vi "Kikusui PLZ-Configure Input.vi"(8 "error in":errorcluster, 9 "Enable Input Short":bool, 10 "Enable Input":bool, 11 "Kikusui PLZ Setting In":T1={"VISA Resource Name"="", "Baud Rate"=19200, "Stop Bits"=20, "Wait For Read(ms)"=0} {"Stop Bits" items=["1.0"=10, "2.0"=20]; "Baud Rate" items=["2400"=2400, "4800"=4800, "9600"=9600, "19200"=19200]}) -> (0 "error out":errorcluster, 3 "Kikusui PLZ Setting Out":T1={"VISA Resource Name"="", "Baud Rate"=19200, "Stop Bits"=20, "Wait For Read(ms)"=0} {"Stop Bits" items=["1.0"=10, "2.0"=20]; "Baud Rate" items=["2400"=2400, "4800"=4800, "9600"=9600, "19200"=19200]})   [LabVIEW 2018]
doc: "Configures the input state and the input short to either on or off."
uses:
  Data Def/Kikusui PLZ-Setting.ctl
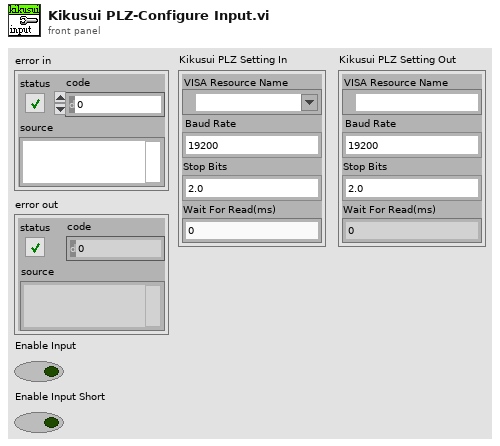
[diagram p1: front panel]
types:
  T1 = typedef "Kikusui PLZ-Setting.ctl" = cluster{"VISA Resource Name":refnum<visa-resource-name>, "Baud Rate":u32, "Stop Bits":u16, "Wait For Read(ms)":u32}
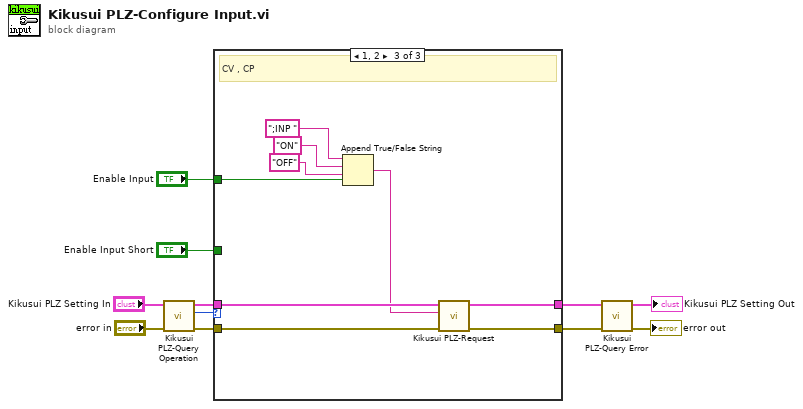
[diagram p0: block diagram]
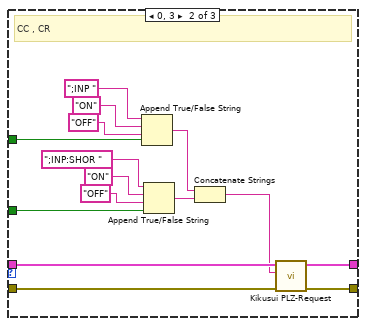
[diagram p3: hidden frame]
diagram:
  n1 = call "Kikusui PLZ-Query Operation.vi"("error in"="error in", "Kikusui PLZ Setting In"="Kikusui PLZ Setting In") -> ("error out"=w4:errorcluster, "Operation Mode"=w3:u16, "Kikusui PLZ Setting Out"=w5:T1)  [unwired: 7 in]
  n2 = case shown="1, 2" w3 {
    tunnel: w5 -> [w13 w17 w30]
    tunnel: w4 -> [w12 w18 w33]
    tunnel: "Enable Input" -> [_ w22 w34]
    tunnel: "Enable Input Short" -> [_ w21 _]
    tunnel: [w12 w15 w32] -> w9
    tunnel: [w13 w16 w31] -> w8
    frame Default {
    }
    frame 0, 3 {
      # "CC , CR"
      n3 = Append True/False String(1:w22, 2:"OFF" ("false string"), 3:"ON" ("true string"), 4:";INP " ("string (\"\")")) -> (0:w19:string)
      n4 = Append True/False String(1:w21, 2:"OFF" ("false string"), 3:"ON" ("true string"), 4:";INP:SHOR " ("string (\"\")")) -> (0:w20:string)
      n5 = Concatenate Strings(w19, w20) -> (w14:string)
      n6 = call "Kikusui PLZ-Request.vi"("error in"=w18, "Command"=w14, "Kikusui PLZ Setting In"=w17) -> ("error out"=w15:errorcluster, "Kikusui PLZ Setting Out"=w16:T1)  [unwired: 6 in, 1 out]
    }
    frame 1, 2 {
      # "CV , CP"
      n7 = Append True/False String(1:w34, 2:"OFF" ("false string"), 3:"ON" ("true string"), 4:";INP " ("string (\"\")")) -> (0:w29:string)
      n8 = call "Kikusui PLZ-Request.vi"("error in"=w33, "Command"=w29, "Kikusui PLZ Setting In"=w30) -> ("error out"=w32:errorcluster, "Kikusui PLZ Setting Out"=w31:T1)  [unwired: 6 in, 1 out]
    }
  }
  n9 = call "Kikusui PLZ-Query Error.vi"("error in"=w9, "Kikusui PLZ Setting In"=w8) -> ("error out"=→"error out":errorcluster, "Kikusui PLZ Setting Out"=→"Kikusui PLZ Setting Out":T1)  [unwired: 8 in]
